vi "lv sample.vi"() -> ()   [LabVIEW 2026]
uses:
  bin/nominalClient_64.dll
panel:
  out "error out":errorcluster
  in  "api token":string
  out "username":string
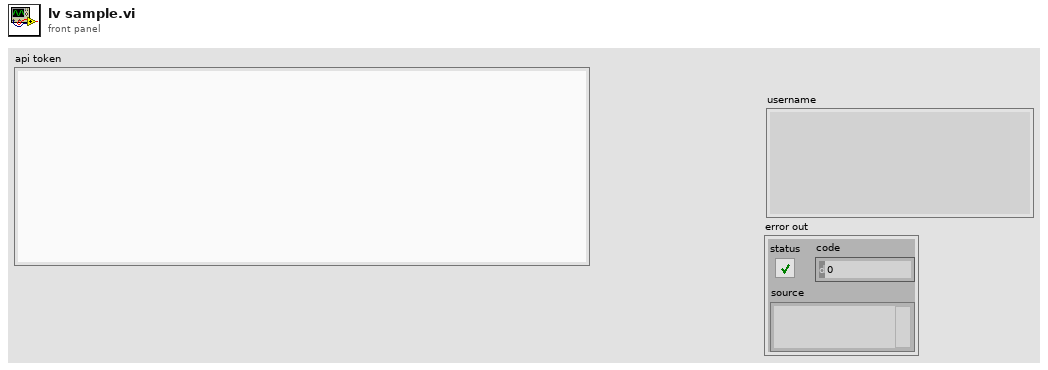
[diagram p1: front panel]
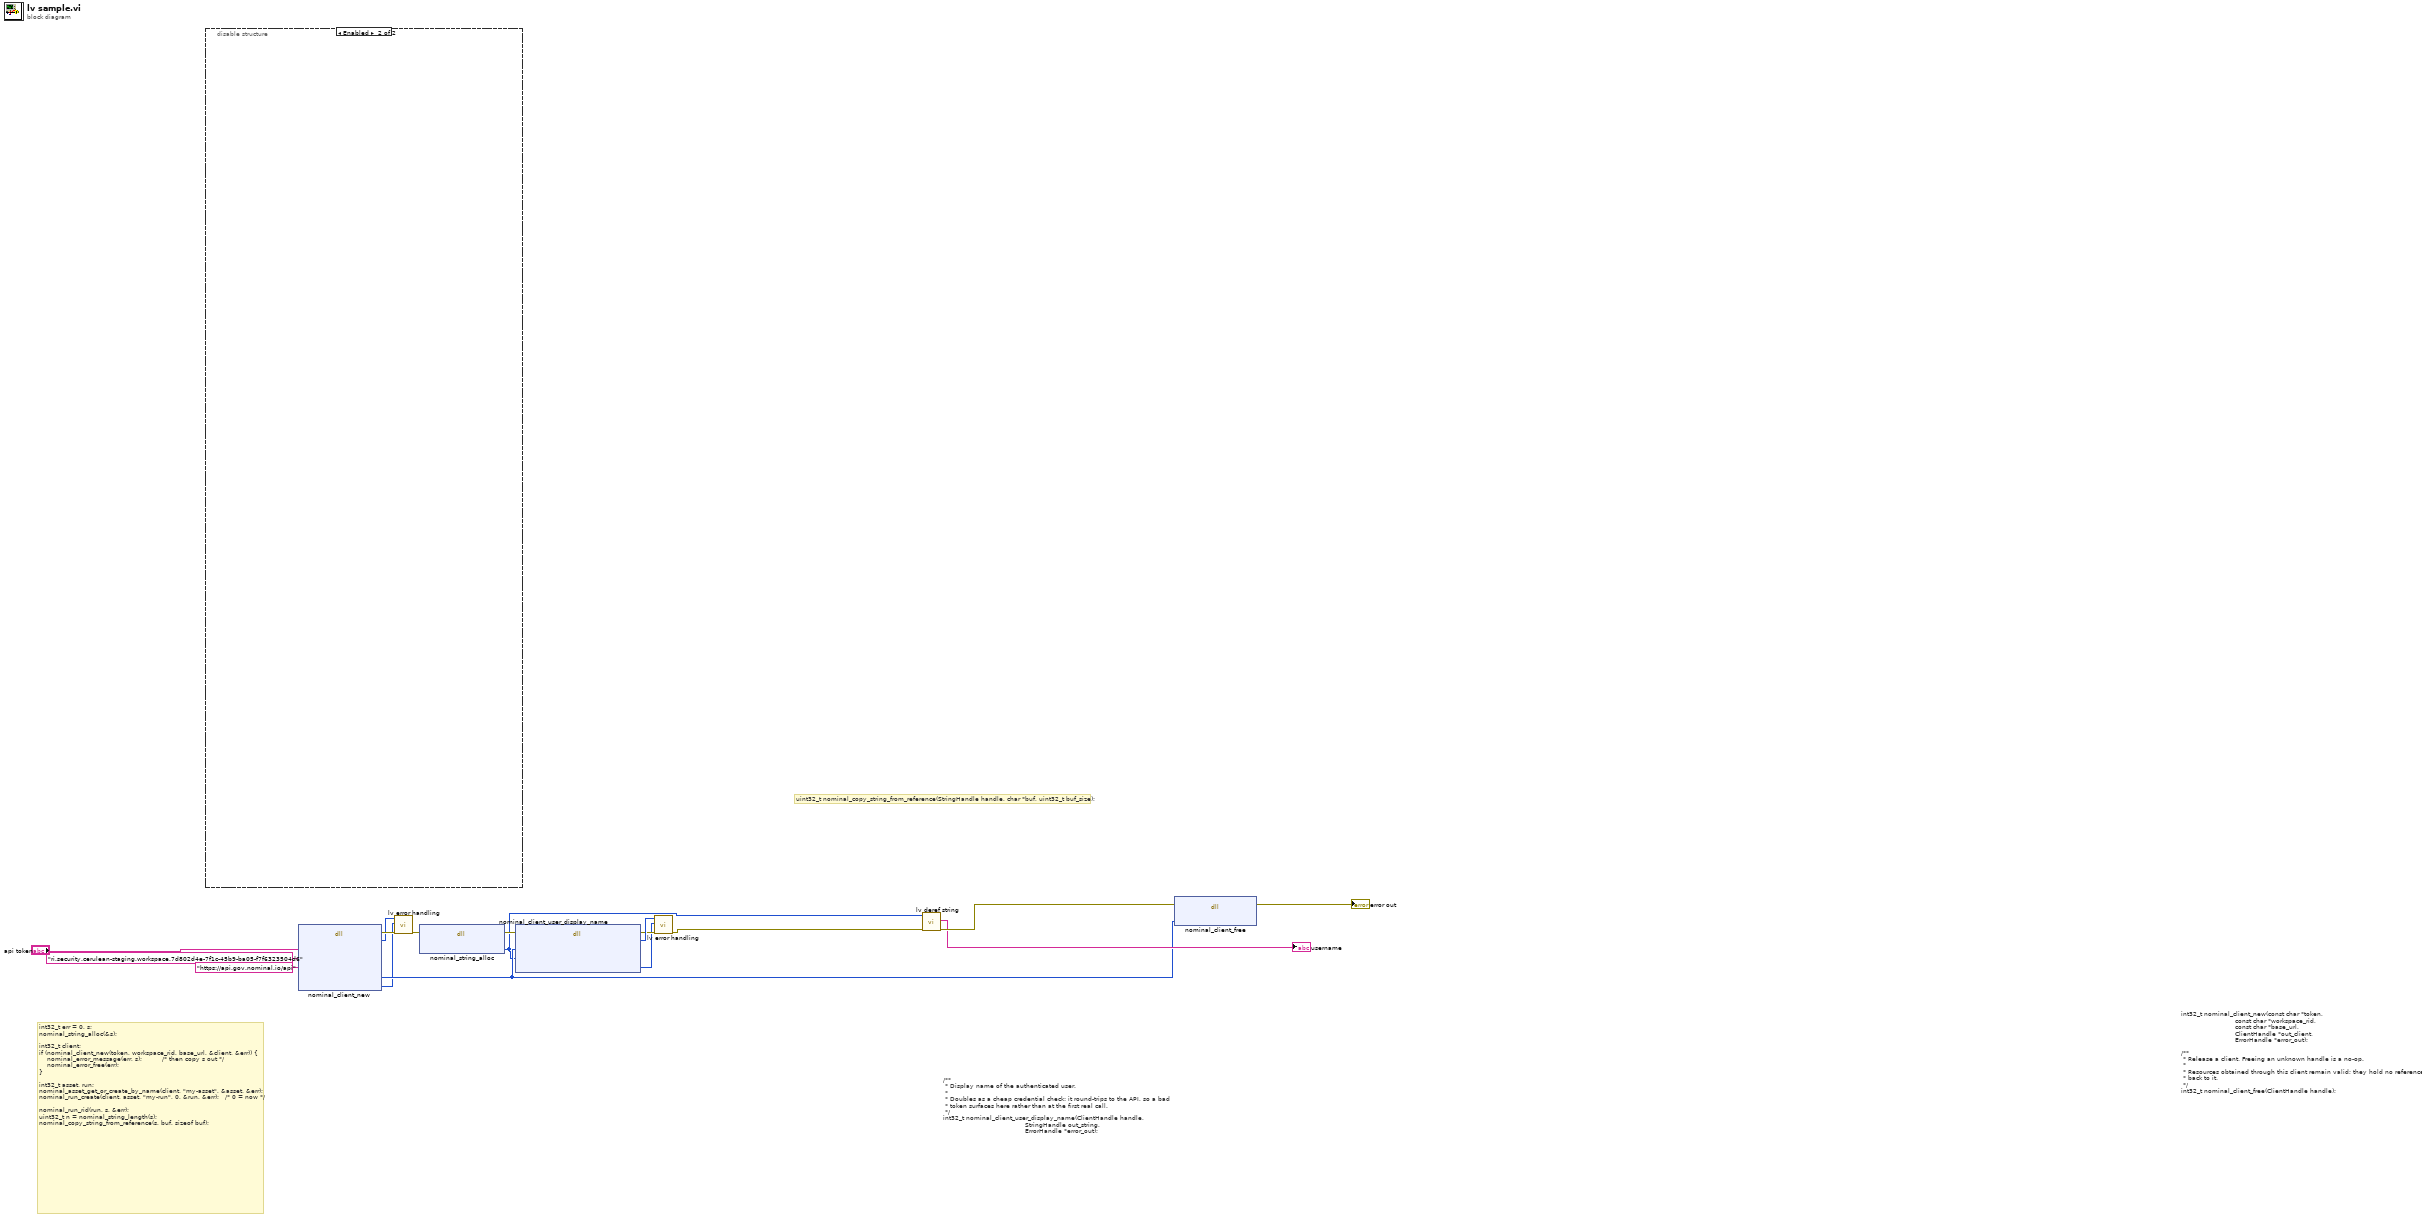
[diagram p0: block diagram]
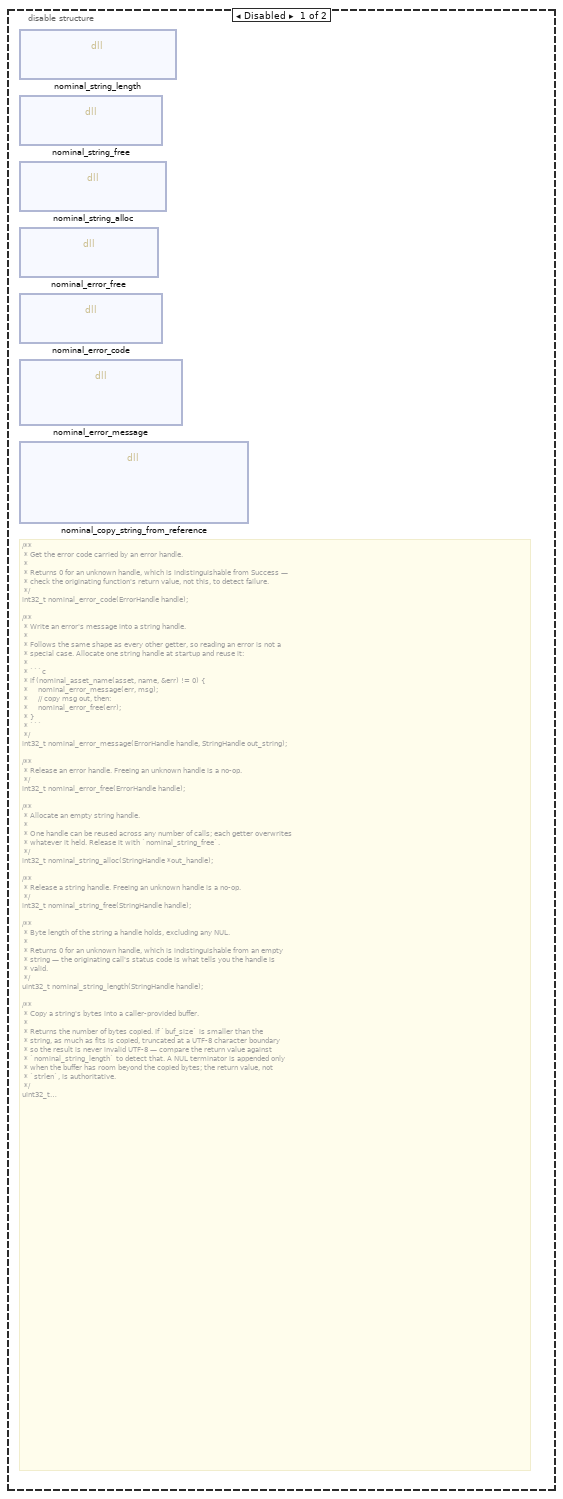
[diagram p2: hidden frame]
diagram:
  # "uint32_t nominal_copy_string_from_reference(StringHandle handle, char *buf, uint32_t buf_size);"
  # "int32_t err = 0, s;\nnominal_string_alloc(&s);\n\nint32_t client;\nif (nominal_client_new(token, workspace_rid, base_url, &client, &err)) {\n    nominal_error_message(err, s);          /* then copy s out */\n    nominal_error_free(err);\n}\n\nint32_t asset, run;\nnominal_asset_get_or_create_by_name(client, \"my-asset\", &asset, &err);\nnominal_run_create(client, asset, \"my-run\", 0, &run, &err);   /* 0 = now */\n\nnominal_run_rid(run, s, &err);\nuint32_t n = nominal_string_length(s);\nnominal_copy_string_from_reference(s, buf, sizeof buf);"
  # "/**\n * Display name of the authenticated user.\n *\n * Doubles as a cheap credential check: it round-trips to the API, so a bad\n * token surfaces here rather than at the first real call.\n */\nint32_t nominal_client_user_display_name(ClientHandle handle,\n                                         StringHandle out_string,\n                                         ErrorHandle *error_out);"
  # "int32_t nominal_client_new(const char *token,\n                           const char *workspace_rid,\n                           const char *base_url,\n                           ClientHandle *out_client,\n                           ErrorHandle *error_out);\n\n/**\n * Release a client. Freeing an unknown handle is a no-op.\n *\n * Resources obtained through this client remain valid; they hold no reference\n * back to it.\n */\nint32_t nominal_client_free(ClientHandle handle);"
  n1 = disable-structure shown="Enabled" {
    frame Disabled {
      # "/**\n * Get the error code carried by an error handle.\n *\n * Returns 0 for an unknown handle, which is indistinguishable from Success —\n * check the originating function's return value, not this, to detect failure.\n */\nint32_t nominal_error_code(ErrorHandle handle);\n\n/**\n * Write an error's message into a string handle.\n *\n * Follows the same shape as every other getter, so reading an error is not a\n * special case. Allocate one string handle at startup and reuse it:\n *\n * ```c\n * if (nominal_asset_name(asset, name, &err) != 0) {\n *     nominal_error_message(err, msg);\n *     // copy msg out, then:\n *     nominal_error_free(err);\n * }\n * ```\n */\nint32_t nominal_error_message(ErrorHandle handle, StringHandle out_string);\n\n/**\n * Release an error handle. Freeing an unknown handle is a no-op.\n */\nint32_t nominal_error_free(ErrorHandle handle);\n\n/**\n * Allocate an empty string handle.\n *\n * One handle can be reused across any number of calls; each getter overwrites\n * whatever it held. Release it with `nominal_string_free`.\n */\nint32_t nominal_string_alloc(StringHandle *out_handle);\n\n/**\n * Release a string handle. Freeing an unknown handle is a no-op.\n */\nint32_t nominal_string_free(StringHandle handle);\n\n/**\n * Byte length of the string a handle holds, excluding any NUL.\n *\n * Returns 0 for an unknown handle, which is indistinguishable from an empty\n * string — the originating call's status code is what tells you the handle is\n * valid.\n */\nuint32_t nominal_string_length(StringHandle handle);\n\n/**\n * Copy a string's bytes into a caller-provided buffer.\n *\n * Returns the number of bytes copied. If `buf_size` is smaller than the\n * string, as much as fits is copied, truncated at a UTF-8 character boundary\n * so the result is never invalid UTF-8 — compare the return value against\n * `nominal_string_length` to detect that. A NUL terminator is appended only\n * when the buffer has room beyond the copied bytes; the return value, not\n * `strlen`, is authoritative.\n */\nuint32_t nominal_copy_string_from_reference(StringHandle handle, char *buf, uint32_t buf_size);"
      n2 = dll-call lib="C:/sw/nominal-c/bin/nominalClient_64.dll" fn="nominal_string_length"() -> ()  [unwired: 6 in, 2 out]
      n3 = dll-call lib="C:/sw/nominal-c/bin/nominalClient_64.dll" fn="nominal_string_free"() -> ()  [unwired: 6 in, 2 out]
      n4 = dll-call lib="C:/sw/nominal-c/bin/nominalClient_64.dll" fn="nominal_string_alloc"() -> ()  [unwired: 6 in, 2 out]
      n5 = dll-call lib="C:/sw/nominal-c/bin/nominalClient_64.dll" fn="nominal_error_free"() -> ()  [unwired: 6 in, 2 out]
      n6 = dll-call lib="C:/sw/nominal-c/bin/nominalClient_64.dll" fn="nominal_error_code"() -> ()  [unwired: 6 in, 2 out]
      n7 = dll-call lib="C:/sw/nominal-c/bin/nominalClient_64.dll" fn="nominal_error_message"() -> ()  [unwired: 8 in, 2 out]
      n8 = dll-call lib="C:/sw/nominal-c/bin/nominalClient_64.dll" fn="nominal_copy_string_from_reference"() -> ()  [unwired: 10 in, 2 out]
    }
    frame Enabled {
    }
  }
  n9 = dll-call lib="C:/sw/nominal-c/bin/nominalClient_64.dll" fn="nominal_client_new"("api token"="api token", "workspace rid"="ri.security.cerulean-staging.workspace.7d802d4e-7f1c-45b9-ba05-f7f6323504d6", "base url"="https://api.gov.nominal.io/api") -> (error out=w17:errorcluster, "return type"=w16:i32, "client handle"=w11:i32, "errorout"=w2:i32)  [unwired: 8 in, 1 out]
  n10 = call "lv error handling.vi"("error in"=w17, "error handle"=w2, "return code"=w16) -> ("error out"=w13:errorcluster)  [unwired: 8 in]
  n11 = dll-call lib="C:/sw/nominal-c/bin/nominalClient_64.dll" fn="nominal_string_alloc"(error in=w13) -> (error out=w15:errorcluster, "string handle"=w4:i32)  [unwired: 4 in, 1 out]
  n12 = dll-call lib="C:/sw/nominal-c/bin/nominalClient_64.dll" fn="nominal_client_user_display_name"(error in=w15, "client handle"=w11, "display name handle"=w4) -> (error out=w9:errorcluster, "return type"=w10:i32, "errorout"=w1:u64)  [unwired: 5 in, 1 out]
  n13 = call "lv error handling.vi"("error in"=w9, "error handle"=w1, "return code"=w10) -> ("error out"=w8:errorcluster)  [unwired: 8 in]
  n14 = call "lv deref string.vi"("error in"=w8, "string handle"=w4) -> ("error out"=w14:errorcluster, "outbuffer"=→"username":string)  [unwired: 8 in]
  n15 = dll-call lib="C:/sw/nominal-c/bin/nominalClient_64.dll" fn="nominal_client_free"(error in=w14, "client handle"=w11) -> (error out=→"error out":errorcluster)  [unwired: 4 in, 1 out]
